vi "SENS_FOM_RANGE_SEGM_BWID_FREQ.vi"(0 "VISA IN":refnum<visa-resource-name>, 1 "Range":i32, 2 "Segment":i32, 3 "IF BW(Hz)":dbl, 5 "error in":errorcluster, 7 "Channel":i32) -> (14 "VISA Out":refnum<visa-resource-name>, 19 "error out":errorcluster)   [LabVIEW 2018, in "PNA-X.lvlib"]
uses:
  PNA-X.lvlib
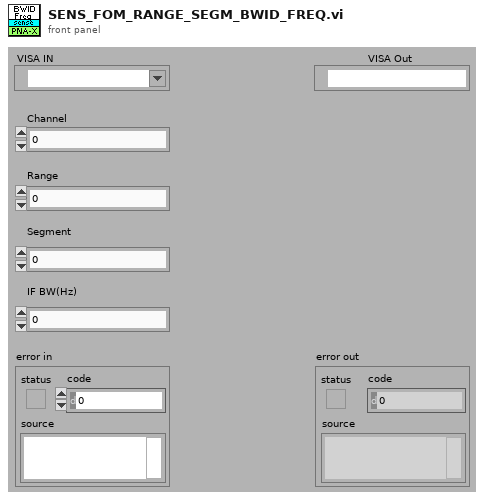
[diagram p1: front panel]
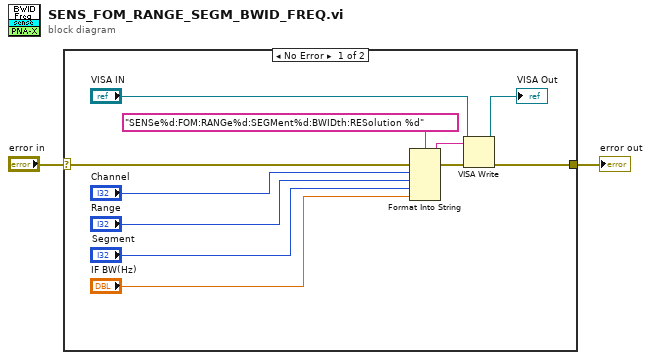
[diagram p0: block diagram]
diagram:
  n1 = case shown="No Error" "error in" {
    selector: "error in" -> [w13 w14]
    tunnel: [w8 w14] -> w1
    frame No Error {
      n2 = Format Into String(format string="SENSe%d:FOM:RANGe%d:SEGMent%d:BWIDth:RESolution %d" ("Cmdline"), error in=w13, "Channel", "Range", "Segment", "IF BW(Hz)") -> (resulting string=w11:string, error out=w12:errorcluster)  [unwired: 1 in]
      n3 = VISA Write(VISA resource name="VISA IN", write buffer=w11, error in (no error)=w12) -> (VISA resource name out=→"VISA Out":refnum<visa-resource-name>, error out=w8:errorcluster)  [unwired: 1 out]
    }
    frame Error {
    }
  }
  "error out" <- w1
